vi "Memory Manager Pre-Build.vi"   [LabVIEW 2017]
uses:
  Build Automation.lvlib
types:
  T1 = cluster{"Status Message":refnum<data-value>, "Progress":refnum<data-value>, "Stop":refnum<data-value>}
  T2 = enum16{"Share clones between instances", "Preallocate clone for each instance"}
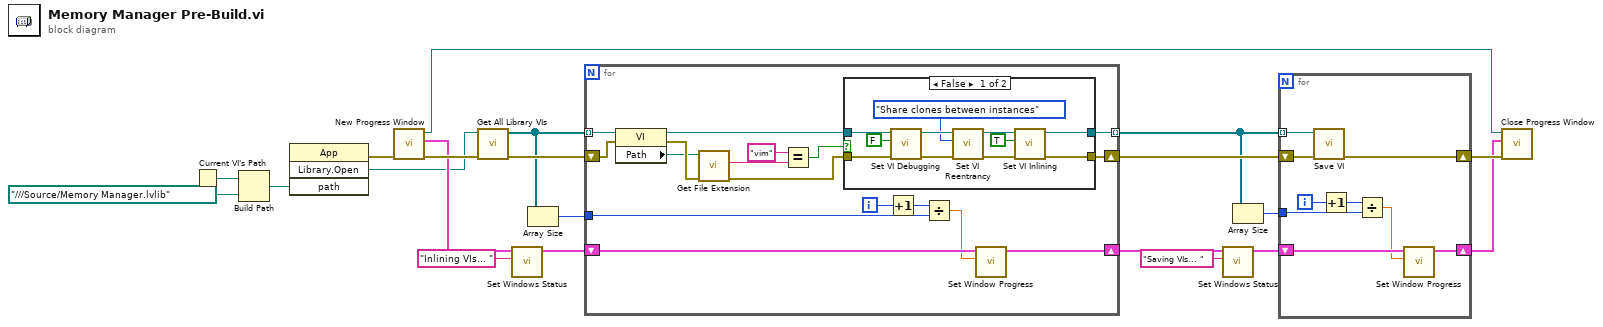
[diagram p0: block diagram]
diagram:
  n1 = Current VI's Path() -> (path=w2:path)
  n2 = Build Path(base path=w2, name or relative path=path "../../../Source/Memory Manager.lvlib" ("stripped path")) -> (appended path=w21:path)
  n3 = invoke class="App" method="Library.Open"("path"=w21) -> (error out=w19:errorcluster, "Open Library"=w8:refnum<vi>)  [unwired: 3 in, 2 out]
  n4 = call "New Progress Window.vi"("error in (no error)"=w19) -> ("error out"=w10:errorcluster, "DVRs"=w9:T1, "VI refnum"=w14:refnum<vi>)  [unwired: 8 in]
  n5 = call "Get All Library VIs.vi"("error in (no error)"=w10, "library ref"=w8) -> ("error out"=w20:errorcluster, "vi refs"=w17:refnum<vi>[])  [unwired: 8 in]
  n6 = call "Set Windows Status.vi"("Status Message"="Inlining VIs... " ("data value"), "DVRs in"=w9) -> ("DVRs out"=w15:T1)  [unwired: 8 in, 1 out]
  n7 = Array Size(array=w17) -> (size(s)=w16:i32)
  n8 = for {
    tunnel: w17 -> [w31] mode=indexing
    shift-right: [w32] -> w13
    shift-left: w20 -> [w30]
    tunnel: w16 -> [w27]
    shift-right: [w34] -> w12
    shift-left: w15 -> [w36]
    tunnel: [w33] -> w6 mode=indexing
    i -> [w38]
    n9 = property class="VI"(reference=w31, error in=w30) -> (reference out=w26:refnum<vi>, error out=w25:errorcluster, "Path"=w22:path)
    n10 = call <vilib>:"Get File Extension.vi"("error in (no error)"=w25, "file"=w22) -> ("error out"=w24:errorcluster, "lowercase file extension"=w23:string)  [unwired: 5 in, 3 out]
    n11 = Equal?(x="vim" ("y"), y=w23) -> (x = y?=w28:bool)
    n12 = case shown="False" w28 {
      tunnel: [w42 w50] -> w33
      tunnel: [w39 w51] -> w32
      tunnel: w24 -> [w41 w51]
      tunnel: w26 -> [w40 w50]
      frame False {
        n13 = call "Set VI Debugging.vi"("error in (no error)"=w41, "Allow Debugging"=FALSE, "vi ref in"=w40) -> ("error out"=w47:errorcluster, "vi ref out"=w48:refnum<vi>)  [unwired: 7 in]
        n14 = call "Set VI Reentrancy.vi"("error in (no error)"=w47, "Reentrancy Type"=T2."Share clones between instances", "vi ref in"=w48) -> ("error out"=w45:errorcluster, "vi ref out"=w46:refnum<vi>)  [unwired: 7 in]
        n15 = call "Set VI Inlining.vi"("error in (no error)"=w45, "Inline VI"=TRUE, "vi ref in"=w46) -> ("error out"=w39:errorcluster, "vi ref out"=w42:refnum<vi>)  [unwired: 7 in]
      }
      frame True {
      }
    }
    n16 = Increment(x=w38) -> (x+1=w37:i32)
    n17 = Divide(x=w37, y=w27) -> (x/y=w35:dbl)
    n18 = call "Set Window Progress.vi"("Progress"=w35, "DVRs in"=w36) -> ("DVRs out"=w34:T1)  [unwired: 8 in, 1 out]
  }
  n19 = call "Set Windows Status.vi"("Status Message"="Saving VIs... ", "DVRs in"=w12) -> ("DVRs out"=w7:T1)  [unwired: 8 in, 1 out]
  n20 = Array Size(array=w6) -> (size(s)=w5:i32)
  n21 = for {
    shift-right: [w58] -> w4
    shift-left: w13 -> [w60]
    tunnel: w6 -> [w59] mode=indexing
    shift-right: [w52] -> w3
    shift-left: w7 -> [w54]
    tunnel: w5 -> [w56]
    i -> [w55]
    n22 = call "Save VI.vi"("error in (no error)"=w60, "vi ref in"=w59) -> ("error out"=w58:errorcluster)  [unwired: 8 in, 1 out]
    n23 = Increment(x=w55) -> (x+1=w57:i32)
    n24 = Divide(x=w57, y=w56) -> (x/y=w53:dbl)
    n25 = call "Set Window Progress.vi"("Progress"=w53, "DVRs in"=w54) -> ("DVRs out"=w52:T1)  [unwired: 8 in, 1 out]
  }
  n26 = call "Close Progress Window.vi"("error in (no error)"=w4, "DVRs in"=w3, "VI refnum"=w14) -> ()  [unwired: 8 in, 1 out]
